vi "add_multi_controls_command.vi"(7 "Numeric":i32, 8 "error in":errorcluster, 9 "Controls Specs":T1[](array[typedef]), 10 "Instrument Command":string, 11 "VI Ref In":refnum<vi>) -> (0 "error out":errorcluster, 3 "VI Ref Out":refnum<vi>)   [LabVIEW 2018]
uses:
  TypeDefinitions/single_control_spec.ctl
  TypeDefinitions/control_data_type.ctl
  TypeDefinitions/control_class.ctl
  TypeDefinitions/ring_string_and_value.ctl
  Iternl/ConttWire/TypeDefines/connect_with_last_node_types.ctl
  Misc/AddNode/TypeDefinitions/node_types.ctl
  Iternl/GetNodeTerm/StringProcessingNode/TypeDefinitions/string_node_type.ctl
  Iternl/CalPos/CmdToStr/TypeDefinitions/main_position_types.ctl
  Iternl/AddObj/AddControl/TypeDefinitions/bd_control_type.ctl
  Iternl/CalPos/ParaToStr/TypeDefinitions/sub_position_type.ctl
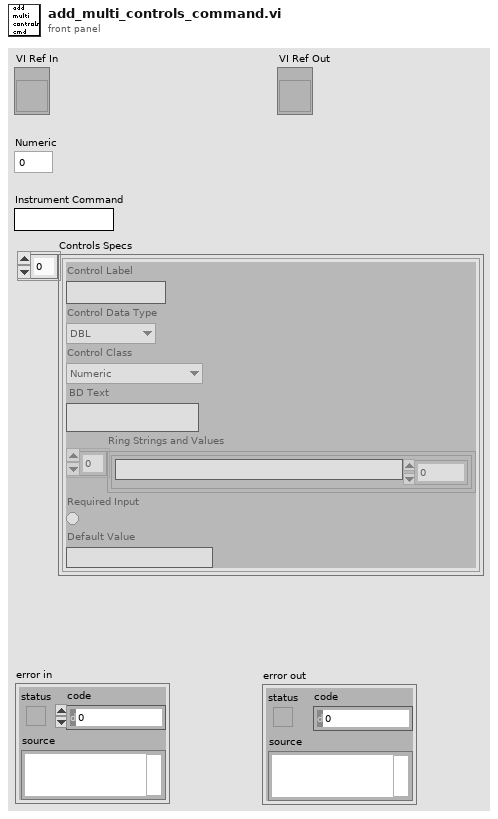
[diagram p1: front panel]
types:
  T1 = typedef "single_control_spec.ctl" = cluster{"Control Label":string, "Control Data Type":T2, "Control Class":T3, "BD Text":string, "Ring Strings and Values":T4[], "Required Input":bool, "Default Value":string}
  T2 = typedef "control_data_type.ctl" = enum16{"DBL", "I32", "Boolean", "String", "U16", "U32", "EXT", "SGL", "I16", "U8", "I8", "I64", "U64", "Waveform", "Reference", "Variant", "Cluster"}
  T3 = typedef "control_class.ctl" = enum16{"Numeric", "Vertical Slide Switch", "Text Ring", "String", "Array", "VISAName", "WaveformGraph", "Cluster"}
  T4 = typedef "ring_string_and_value.ctl" = cluster{"String":string, "Value":dbl}
  T5 = enum16{"Node", "FormatNodeForMultipleControls", "BoolConstant", "FormatConstant", "1stSubNodeX"}
  T6 = typedef "main_position_types.ctl" = enum16{"Node", "FormatNodeForMultipleControls", "BoolConstant", "FormatConstant", "1stSubNodeX"}
  T7 = typedef "string_node_type.ctl" = enum16{"FormatIntoString", "PickLine", "AppendTrueFalse", "ConcatenateStrings"}
  T8 = typedef "node_types.ctl" = enum16{"FormatIntoString", "PickLine", "AppendTrueFalse", "VISAWrite", "SubVI", "ConcatenateStrings", "VISARead", "ProperyNode", "ScanFromString", "SpreadSheetStringToArray"}
  T9 = typedef "sub_position_type.ctl" = enum16{"BoolNode", "BoolConst", "RingConstNode", "Numeri/String"}
  T10 = typedef "bd_control_type.ctl" = enum16{"Numeric", "Ring", "Boolean", "String", "VisaIn", "VisaOut", "Error In", "Error Out", "Array", "Waveform"}
  T11 = typedef "connect_with_last_node_types.ctl" = u16
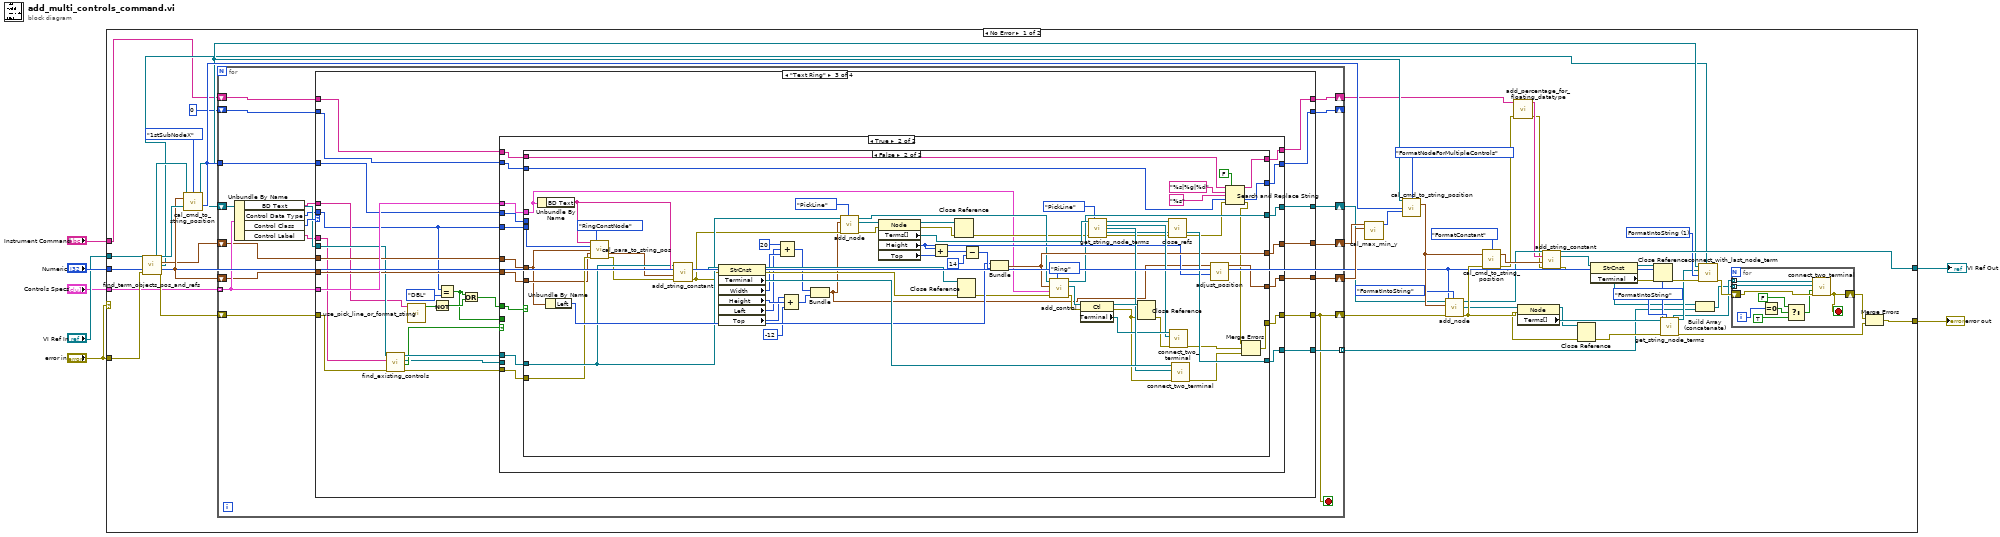
[diagram p0: block diagram]
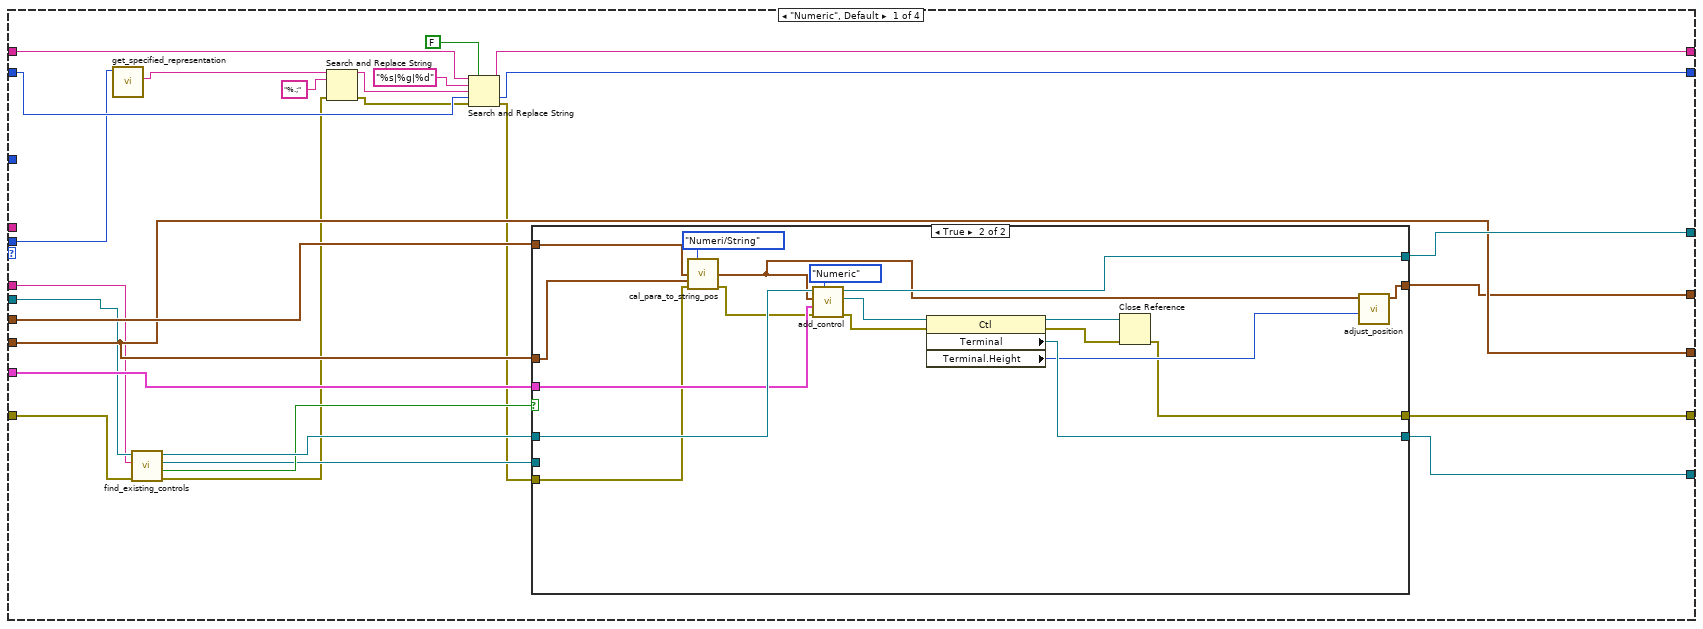
[diagram p2: hidden frame]
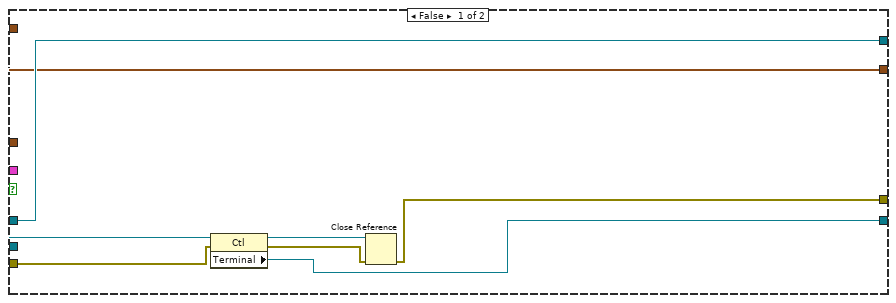
[diagram p3: hidden frame]
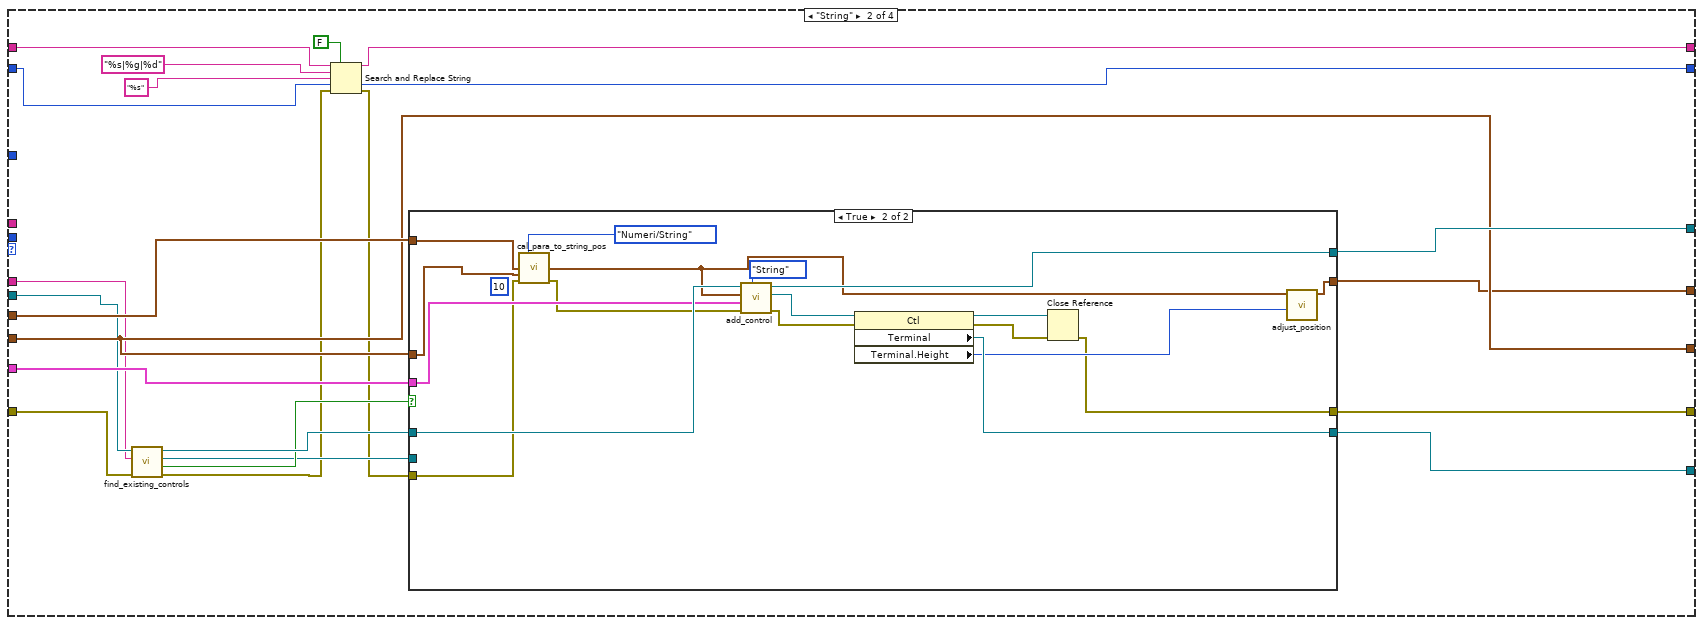
[diagram p4: hidden frame]
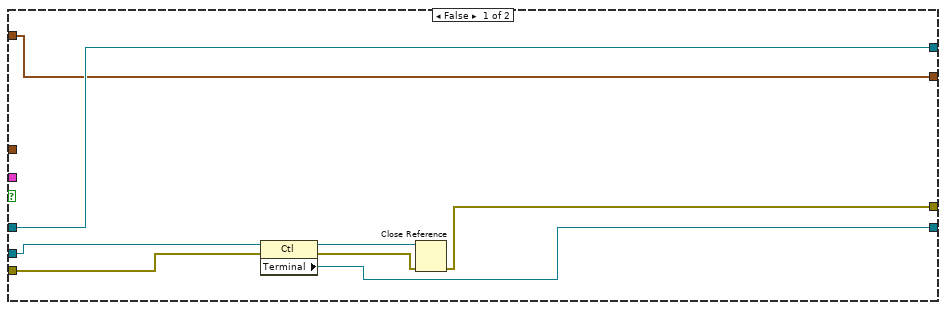
[diagram p5: hidden frame]
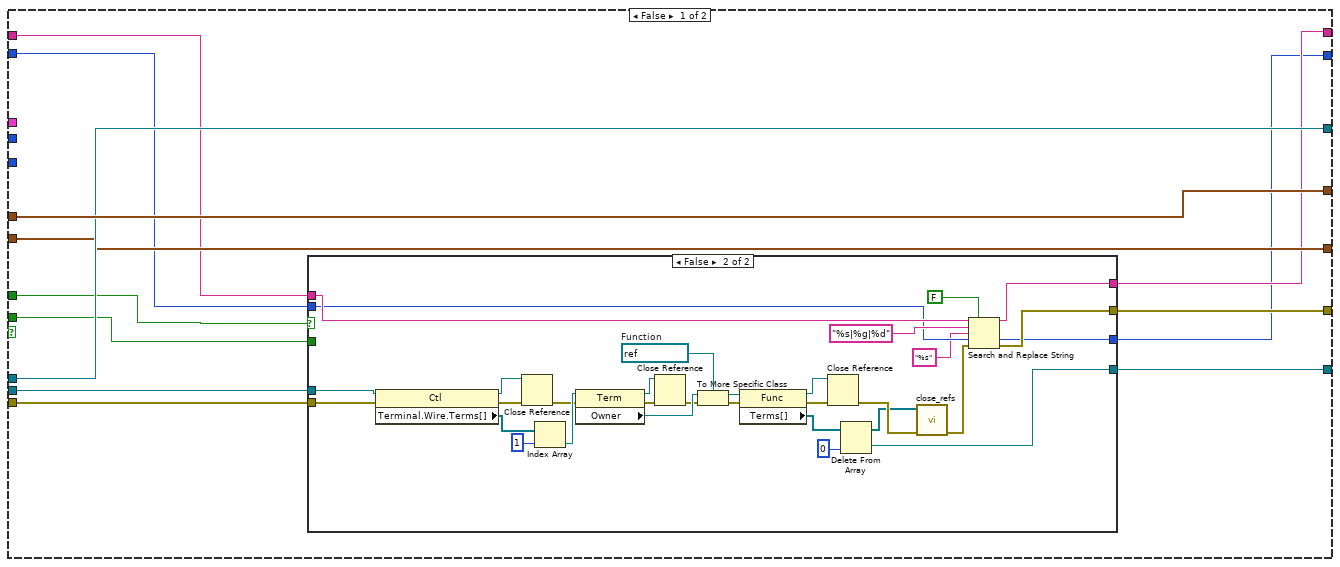
[diagram p6: hidden frame]
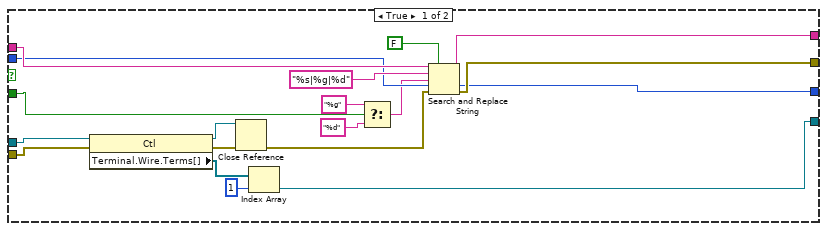
[diagram p7: hidden frame]
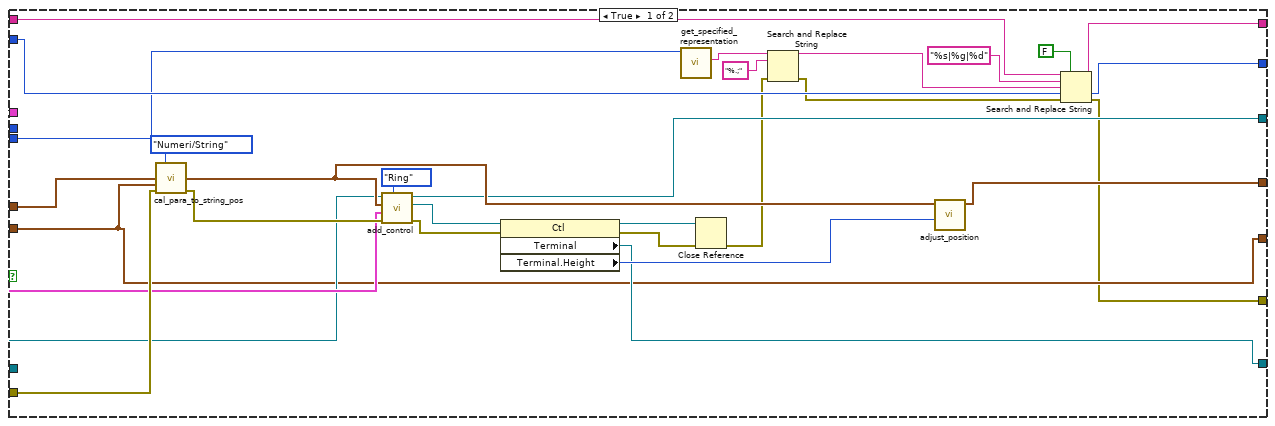
[diagram p8: hidden frame]
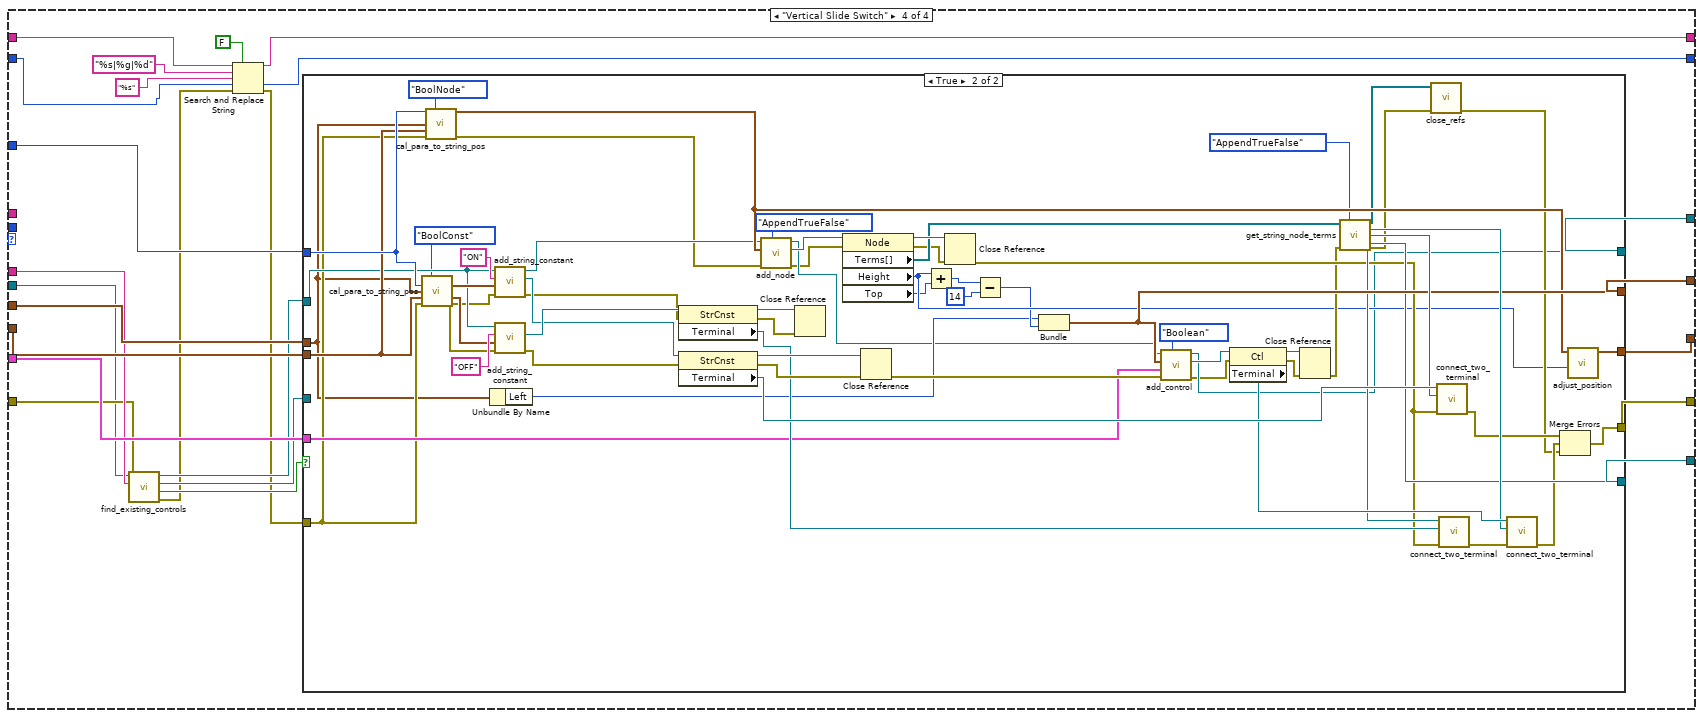
[diagram p9: hidden frame]
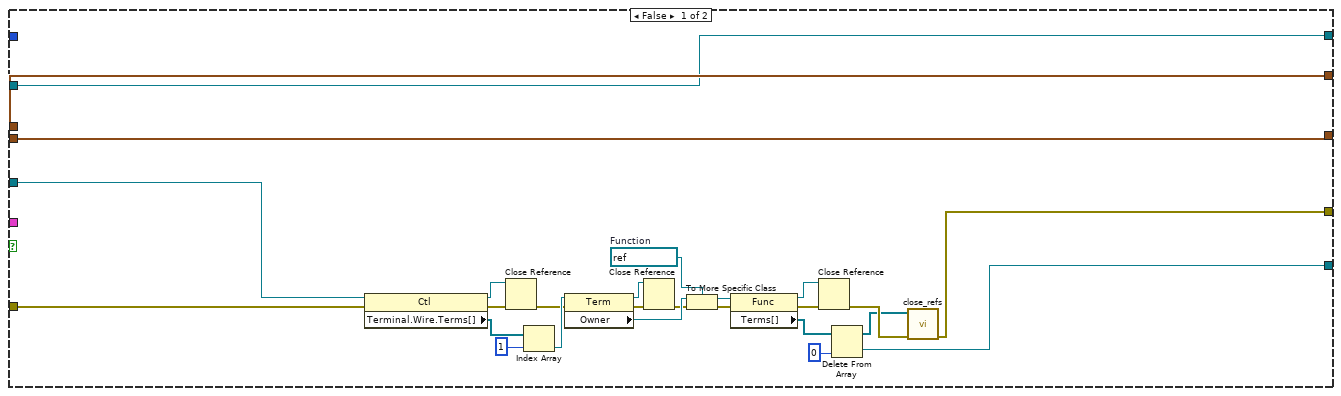
[diagram p10: hidden frame]
diagram:
  n1 = case shown="No Error" "error in" {
    tunnel: [w49 w506] -> w7
    tunnel: [w48 w507] -> w6
    tunnel: "error in" -> [w40 w507]
    tunnel: "Numeric" -> [w31 _]
    tunnel: "Instrument Command" -> [w13 _]
    tunnel: "VI Ref In" -> [w16 w506]
    tunnel: "Controls Specs" -> [w15 _]
    frame No Error {
      w34 = T11 1 items=["AppendTrueFalseString"=4, "PickLine"=3, "FormatIntoString"=1] ("Terminal Index")
      n2 = call "find_term_objects_pos_and_refs.vi"("VI Ref In"=w16, "error in (no error)"=w40) -> ("Last Function"=w38:refnum<vi>, "VI Ref Out"=w36:refnum<vi>, "Last Control Position"=w17:cluster{"Left":i32, "Top":i32}, "Last StrCnst Refnum"=w14:refnum<vi>, "Last Function Position"=w18:cluster{"Left":i32, "Top":i32}, "error out"=w41:errorcluster)  [unwired: 8 out]
      n3 = call "cal_cmd_to_string_position.vi"("Last Function Ref In"=w38, "Enum"=T5."1stSubNodeX", "Main Node BD Position"=w18) -> ("Last Function Ref Out"=w39:refnum<vi>, "1st sub node x position"=w56:i32)  [unwired: 4 in, 7 out]
      n4 = for {
        tunnel: w15 -> [w88] mode=indexing
        shift-right: [w85] -> w19
        shift-left: w36 -> [w86]
        tunnel: [w84] -> w25 mode=indexing
        shift-right: [w83] -> w58
        shift-left: w17 -> [w81]
        shift-right: [w80] -> w59
        shift-left: w18 -> [w82]
        tunnel: w56 -> [w79]
        shift-right: [w76] -> w42
        shift-left: w41 -> [w78]
        shift-right: [w73] -> w11
        shift-left: w13 -> [w75]
        shift-right: [w72] -> _
        shift-left: 0 -> [w74]
        stop <- w76 stop-if-true
        n5 = Unbundle By Name(w88) -> ("BD Text"=w70:string, "Control Data Type"=w71:T2, "Control Class"=w87:T3, "Control Label"=w77:string)
        n6 = case shown="\"Text Ring\"" w87 {
          tunnel: w88 -> [w114 w162 w215 w416]
          tunnel: w86 -> [w107 w155 w207 w404]
          tunnel: [w113 w161 w213 w415] -> w85
          tunnel: [w112 w160 w214 w413] -> w84
          tunnel: [w109 w157 w211 w414] -> w83
          tunnel: w82 -> [w110 w158 w209 w411]
          tunnel: w81 -> [w111 w159 w208 w412]
          tunnel: [w110 w158 w212 w410] -> w80
          tunnel: w79 -> [_ _ w210 w409]
          tunnel: w78 -> [w105 w153 w201 w406]
          tunnel: [w108 w156 w189 w408] -> w76
          tunnel: w77 -> [w106 w154 w204 w407]
          tunnel: w75 -> [w101 w143 w200 w395]
          tunnel: w74 -> [w99 w146 w199 w398]
          tunnel: [w89 w142 w198 w394] -> w73
          tunnel: [w90 w141 w197 w393] -> w72
          tunnel: w71 -> [w94 _ w194 _]
          tunnel: w70 -> [_ _ w196 _]
          frame "Numeric", Default {
            n7 = call "get_specified_representation.vi"("Control Data Type"=w94) -> ("Format String"=w96:string)  [unwired: 10 out]
            n8 = call "find_existing_controls.vi"("error in (no error)"=w105, "Label Text"=w106, "VI Ref In"=w107) -> ("error out"=w92:errorcluster, "New Ctrl"=w103:bool, "Ctrl Ref Out"=w102:refnum<vi>, "VI Ref Out"=w104:refnum<vi>)  [unwired: 5 out]
            n9 = Search and Replace String(input string=w96, search string="%.;", error in=w92) -> (result string=w93:string, error out=w91:errorcluster)  [unwired: 7 out]
            n10 = Search and Replace String(replace all?=FALSE ("replace all? (F)"), input string=w101, search string="%s|%g|%d", replace string=w93, offset=w99, error in=w91) -> (result string=w89:string, offset past replacement=w90:i32, error out=w97:errorcluster)  [unwired: 3 out]
            n11 = case shown="True" w103 {
              tunnel: w114 -> [_ w130]
              tunnel: [w120 w140] -> w113
              tunnel: [w116 w137] -> w112
              tunnel: w111 -> [w119 w128]
              tunnel: w110 -> [_ w127]
              tunnel: [w119 w133] -> w109
              tunnel: [w115 w132] -> w108
              tunnel: w97 -> [w121 w126]
              tunnel: w104 -> [w120 w131]
              tunnel: w102 -> [w122 _]
              frame False {
                n12 = property class="Ctl"(reference=w122, error in=w121) -> (reference out=w117:refnum<vi>, error out=w118:errorcluster, "Terminal"=w116:refnum<vi>)
                n13 = Close Reference(reference=w117, error in (no error)=w118) -> (error out=w115:errorcluster)
              }
              frame True {
                n14 = call "cal_para_to_string_pos.vi"("Enum"=sub_position_type."Numeri/String", "Last Control Position"=w128, "Last Function  Position"=w127, "error in"=w126) -> ("Control BD Position"=w125:cluster{"1st sub node x position":i32, i32}, "error out"=w124:errorcluster)  [unwired: 2 in, 8 out]
                n15 = call "add_control.vi"("Add Control Type"=bd_control_type."Numeric" ("Enum"), "error in (no error)"=w124, "Single Control Spec"=w130, "BD Position"=w125, "VI Ref In"=w131) -> ("error out"=w135:errorcluster, "Control Ref Out"=w139:refnum<vi>, "VI Ref Out"=w140:refnum<vi>)  [unwired: 4 out]
                n16 = property class="Ctl"(reference=w139, error in=w135) -> (reference out=w138:refnum<vi>, error out=w136:errorcluster, "Terminal"=w137:refnum<vi>, "Terminal.Height"=w134:u32)
                n17 = Close Reference(reference=w138, error in (no error)=w136) -> (error out=w132:errorcluster)
                n18 = call "adjust_position.vi"("Y Offset"=w134, "Position In"=w125) -> ("Position Out"=w133:cluster{"Left":i32, "Top":i32})  [unwired: 1 in, 8 out]
              }
            }
          }
          frame "String" {
            n19 = call "find_existing_controls.vi"("error in (no error)"=w153, "Label Text"=w154, "VI Ref In"=w155) -> ("error out"=w145:errorcluster, "New Ctrl"=w151:bool, "Ctrl Ref Out"=w150:refnum<vi>, "VI Ref Out"=w152:refnum<vi>)  [unwired: 5 out]
            n20 = Search and Replace String(replace all?=FALSE ("replace all? (F)"), input string=w143, search string="%s|%g|%d", replace string="%s" ("replace string (\"\")"), offset=w146, error in=w145) -> (result string=w142:string, offset past replacement=w141:i32, error out=w144:errorcluster)  [unwired: 3 out]
            n21 = case shown="True" w151 {
              tunnel: w162 -> [_ w178]
              tunnel: [w168 w188] -> w161
              tunnel: [w164 w185] -> w160
              tunnel: w159 -> [w167 w173]
              tunnel: w158 -> [_ w172]
              tunnel: [w167 w181] -> w157
              tunnel: [w163 w180] -> w156
              tunnel: w144 -> [w169 w175]
              tunnel: w152 -> [w168 w179]
              tunnel: w150 -> [w170 _]
              frame False {
                n22 = property class="Ctl"(reference=w170, error in=w169) -> (reference out=w165:refnum<vi>, error out=w166:errorcluster, "Terminal"=w164:refnum<vi>)
                n23 = Close Reference(reference=w165, error in (no error)=w166) -> (error out=w163:errorcluster)
              }
              frame True {
                (unwired) 10 ("y")
                n24 = call "cal_para_to_string_pos.vi"("Enum"=sub_position_type."Numeri/String", "Last Control Position"=w173, "Last Function  Position"=w172, "error in"=w175) -> ("Control BD Position"=w171:cluster{"1st sub node x position":i32, i32}, "error out"=w174:errorcluster)  [unwired: 2 in, 8 out]
                n25 = call "add_control.vi"("Add Control Type"=bd_control_type."String" ("Enum"), "error in (no error)"=w174, "Single Control Spec"=w178, "BD Position"=w171, "VI Ref In"=w179) -> ("error out"=w183:errorcluster, "Control Ref Out"=w187:refnum<vi>, "VI Ref Out"=w188:refnum<vi>)  [unwired: 4 out]
                n26 = property class="Ctl"(reference=w187, error in=w183) -> (reference out=w186:refnum<vi>, error out=w184:errorcluster, "Terminal"=w185:refnum<vi>, "Terminal.Height"=w182:u32)
                n27 = Close Reference(reference=w186, error in (no error)=w184) -> (error out=w180:errorcluster)
                n28 = call "adjust_position.vi"("Y Offset"=w182, "Position In"=w171) -> ("Position Out"=w181:cluster{"Left":i32, "Top":i32})  [unwired: 1 in, 8 out]
              }
            }
          }
          frame "Text Ring" {
            n29 = call "find_existing_controls.vi"("error in (no error)"=w201, "Label Text"=w204, "VI Ref In"=w207) -> ("error out"=w205:errorcluster, "New Ctrl"=w203:bool, "Ctrl Ref Out"=w202:refnum<vi>, "VI Ref Out"=w206:refnum<vi>)  [unwired: 5 out]
            n30 = call "use_pick_line_or_format_stirng.vi"("BD"=w196) -> ("Pick Line Node?"=w193:bool)  [unwired: 10 out]
            n31 = Not(x=w193) -> (.not. x?=w192:bool)
            n32 = Equal?(x=w194, y=control_data_type."DBL") -> (x = y?=w190:bool)
            n33 = Or(x=w190, y=w192) -> (x .or. y?=w191:bool)
            n34 = case shown="True" w203 {
              tunnel: w215 -> [_ w286]
              tunnel: [w222 w295] -> w214
              tunnel: [w227 w288] -> w213
              tunnel: [w226 w294] -> w212
              tunnel: [w228 w293] -> w211
              tunnel: w210 -> [_ w291]
              tunnel: w209 -> [w226 w287]
              tunnel: w208 -> [w228 w285]
              tunnel: [w225 w292] -> w189
              tunnel: w206 -> [w227 w290]
              tunnel: w205 -> [w223 w289]
              tunnel: w202 -> [w224 _]
              tunnel: w194 -> [_ w279]
              tunnel: w200 -> [w221 w283]
              tunnel: w199 -> [w220 w282]
              tunnel: [w219 w280] -> w198
              tunnel: [w218 w281] -> w197
              tunnel: w191 -> [w217 w284]
              tunnel: w190 -> [w216 _]
              frame False {
                n35 = case shown="False" w217 {
                  tunnel: [w231 w251] -> w225
                  tunnel: w224 -> [w244 w259]
                  tunnel: w223 -> [w243 w258]
                  tunnel: [w241 w257] -> w222
                  tunnel: w221 -> [w238 w254]
                  tunnel: w216 -> [w236 _]
                  tunnel: w220 -> [w237 w253]
                  tunnel: [w229 w249] -> w219
                  tunnel: [w230 w248] -> w218
                  frame True {
                    n36 = property class="Ctl"(reference=w244, error in=w243) -> (reference out=w242:refnum<vi>, error out=w247:errorcluster, "Terminal.Wire.Terms[]"=w246:refnum<vi>[])
                    n37 = Close Reference(reference=w242, error in (no error)=w247) -> (error out=w232:errorcluster)
                    n38 = Index Array(array=w246, index=1) -> (element=w241:refnum<vi>)
                    n39 = Select(t="%g", s=w236, f="%d" ("replace string (\"\")")) -> (s? t:f=w233:string)
                    n40 = Search and Replace String(replace all?=FALSE ("replace all? (F)"), input string=w238, search string="%s|%g|%d", replace string=w233, offset=w237, error in=w232) -> (result string=w229:string, offset past replacement=w230:i32, error out=w231:errorcluster)  [unwired: 3 out]
                  }
                  frame False {
                    w271 = refnum<vi> refnum  # Function
                    n41 = property class="Ctl"(reference=w259, error in=w258) -> (reference out=w270:refnum<vi>, error out=w269:errorcluster, "Terminal.Wire.Terms[]"=w276:refnum<vi>[])
                    n42 = Close Reference(reference=w270, error in (no error)=w269) -> (error out=w266:errorcluster)
                    n43 = Index Array(array=w276, index=1) -> (element=w277:refnum<vi>)
                    n44 = property class="Term"(reference=w277, error in=w266) -> (reference out=w268:refnum<vi>, error out=w267:errorcluster, "Owner"=w272:refnum<vi>)
                    n45 = Close Reference(reference=w268, error in (no error)=w267) -> (error out=w265:errorcluster)
                    n46 = To More Specific Class(target class=w271, reference=w272, error in=w265) -> (specific class reference=w275:refnum<vi>, error out=w273:errorcluster)
                    n47 = property class="Func"(reference=w275, error in=w273) -> (reference out=w262:refnum<vi>, error out=w264:errorcluster, "Terms[]"=w261:refnum<vi>[])
                    n48 = Close Reference(reference=w262, error in (no error)=w264) -> (error out=w263:errorcluster)
                    n49 = Delete From Array(array=w261, index=0) -> (deleted portion=w257:refnum<vi>, array with subset deleted=w260:refnum<vi>[])  [unwired: 1 in]
                    n50 = call "close_refs.vi"("error in"=w263, "Refs[]  In"=w260) -> ("error out"=w252:errorcluster)  [unwired: 9 out]
                    n51 = Search and Replace String(replace all?=FALSE ("replace all? (F)"), input string=w254, search string="%s|%g|%d", replace string="%s" ("replace string (\"\")"), offset=w253, error in=w252) -> (result string=w249:string, offset past replacement=w248:i32, error out=w251:errorcluster)  [unwired: 3 out]
                  }
                }
              }
              frame True {
                n52 = case shown="False" w284 {
                  tunnel: [w311 w379] -> w295
                  tunnel: [w309 w377] -> w294
                  tunnel: [w310 w376] -> w293
                  tunnel: [w304 w375] -> w292
                  tunnel: w291 -> [_ w374]
                  tunnel: w290 -> [w313 w365]
                  tunnel: w289 -> [w315 w363]
                  tunnel: [w312 w357] -> w288
                  tunnel: w287 -> [w309 w356]
                  tunnel: w286 -> [w314 w349]
                  tunnel: w285 -> [w316 w345]
                  tunnel: w283 -> [w306 w333]
                  tunnel: w282 -> [w305 w331]
                  tunnel: [w303 w328] -> w281
                  tunnel: [w302 w327] -> w280
                  tunnel: w279 -> [w299 _]
                  frame True {
                    n53 = call "cal_para_to_string_pos.vi"("Enum"=sub_position_type."Numeri/String", "Last Control Position"=w316, "Last Function  Position"=w309, "error in"=w315) -> ("Control BD Position"=w323:cluster{"1st sub node x position":i32, i32}, "error out"=w324:errorcluster)  [unwired: 2 in, 8 out]
                    n54 = call "add_control.vi"("Add Control Type"=bd_control_type."Ring" ("Enum"), "error in (no error)"=w324, "Single Control Spec"=w314, "BD Position"=w323, "VI Ref In"=w313) -> ("error out"=w320:errorcluster, "Control Ref Out"=w317:refnum<vi>, "VI Ref Out"=w312:refnum<vi>)  [unwired: 4 out]
                    n55 = property class="Ctl"(reference=w317, error in=w320) -> (reference out=w318:refnum<vi>, error out=w319:errorcluster, "Terminal"=w311:refnum<vi>, "Terminal.Height"=w321:u32)
                    n56 = call "get_specified_representation.vi"("Control Data Type"=w299) -> ("Format String"=w301:string)  [unwired: 10 out]
                    n57 = Close Reference(reference=w318, error in (no error)=w319) -> (error out=w298:errorcluster)
                    n58 = Search and Replace String(input string=w301, search string="%.;", error in=w298) -> (result string=w296:string, error out=w297:errorcluster)  [unwired: 7 out]
                    n59 = call "adjust_position.vi"("Y Offset"=w321, "Position In"=w323) -> ("Position Out"=w310:cluster{"Left":i32, "Top":i32})  [unwired: 1 in, 8 out]
                    n60 = Search and Replace String(replace all?=FALSE ("replace all? (F)"), input string=w306, search string="%s|%g|%d", replace string=w296, offset=w305, error in=w297) -> (result string=w302:string, offset past replacement=w303:i32, error out=w304:errorcluster)  [unwired: 3 out]
                  }
                  frame False {
                    n61 = Unbundle By Name(w349) -> ("BD Text"=w370:string)
                    n62 = Unbundle By Name(w345) -> ("Left"=w366:i32)
                    n63 = call "cal_para_to_string_pos.vi"("Bool Disable Command"=w370, "Enum"=sub_position_type."RingConstNode", "1st sub node x position"=w374, "Last Control Position"=w345, "Last Function  Position"=w356, "error in"=w363) -> ("BD Constant Position/Disable String Position"=w326:cluster{"1st sub node x position":i32, i32}, "error out"=w360:errorcluster)  [unwired: 8 out]
                    n64 = call "add_string_constant.vi"("error in"=w360, "BD Position"=w326, "StringConstantValue"=w370, "VI Ref In"=w365) -> ("error out"=w362:errorcluster, "StrCnst Refnum"=w373:refnum<vi>)  [unwired: 6 out]
                    n65 = property class="StrCnst"(reference=w373, error in=w362) -> (reference out=w392:refnum<vi>, error out=w378:errorcluster, "Terminal"=w383:refnum<vi>, "Width"=w344:u32, "Height"=w342:u32, "Left"=w338:i32, "Top"=w337:i32)
                    n66 = Compound Arithmetic op=ADD(20 ("value"), w338, w344) -> (w340:u32)
                    n67 = Compound Arithmetic op=ADD(w337, w342, -12 ("value")) -> (w339:u32)
                    n68 = Bundle(w340, w339) -> (w336:cluster{u32, u32})  [unwired: 1 out]
                    n69 = call "add_node.vi"("Node Type"=node_types."PickLine" ("Enum"), "error in (no error)"=w362, "BD Position"=w336, "VI Ref In"=w365) -> ("error out"=w361:errorcluster, "Node Refnum"=w391:refnum<vi>, "VI Ref Out"=w358:refnum<vi>)  [unwired: 2 in, 3 out]
                    n70 = property class="Node"(reference=w391, error in=w361) -> (reference out=w387:refnum<vi>, error out=w386:errorcluster, "Terms[]"=w385:refnum<vi>[], "Height"=w372:u32, "Top"=w371:i32)
                    n71 = Add(x=w372, y=w371) -> (x+y=w369:u32)
                    n72 = Close Reference(reference=w387, error in (no error)=w386) -> (error out=w352:errorcluster)
                    n73 = Close Reference(reference=w392, error in (no error)=w378) -> (error out=w359:errorcluster)
                    n74 = Subtract(x=w369, y=u32 14) -> (x-y=w367:u32)
                    n75 = Bundle("Left"=w366, w367) -> (w376:cluster{"Left":i32, u32})  [unwired: 1 out]
                    n76 = call "add_control.vi"("Add Control Type"=bd_control_type."Ring" ("Enum"), "error in (no error)"=w359, "Single Control Spec"=w349, "BD Position"=w376, "VI Ref In"=w358) -> ("error out"=w389:errorcluster, "Control Ref Out"=w390:refnum<vi>, "VI Ref Out"=w357:refnum<vi>)  [unwired: 4 out]
                    n77 = property class="Ctl"(reference=w390, error in=w389) -> (reference out=w388:refnum<vi>, error out=w355:errorcluster, "Terminal"=w381:refnum<vi>)
                    n78 = call "get_string_node_terms.vi"("Terms[] In"=w385, "Node Type"=string_node_type."PickLine", "error in (no error)"=w352) -> ("Terms[]  Out"=w384:refnum<vi>[], "Pick Term"=w380:refnum<vi>, "Multiline Term/Enable Term/Concantenate Term"=w382:refnum<vi>, "Pick Line Output Term/Disable Term"=w379:refnum<vi>, "error out"=w351:errorcluster)  [unwired: 1 in, 7 out]
                    n79 = Close Reference(reference=w388, error in (no error)=w355) -> (error out=w364:errorcluster)
                    n80 = call "close_refs.vi"("error in"=w351, "Refs[]  In"=w384) -> ("error out"=w330:errorcluster)  [unwired: 9 out]
                    n81 = call "connect_two_terminal.vi"("error in"=w364, "Terminal 2"=w380, "Terminal 1"=w381) -> ("error out"=w354:errorcluster)  [unwired: 1 in, 7 out]
                    n82 = call "connect_two_terminal.vi"("error in"=w355, "Terminal 2"=w382, "Terminal 1"=w383) -> ("error out"=w353:errorcluster)  [unwired: 1 in, 7 out]
                    n83 = call "adjust_position.vi"("Y Offset"=w372, "Position In"=w336) -> ("Position Out"=w377:cluster{"Left":i32, "Top":i32})  [unwired: 1 in, 8 out]
                    n84 = Search and Replace String(replace all?=FALSE ("replace all? (F)"), input string=w333, search string="%s|%g|%d", replace string="%s" ("replace string (\"\")"), offset=w331, error in=w330) -> (result string=w327:string, offset past replacement=w328:i32, error out=w329:errorcluster)  [unwired: 3 out]
                    n85 = Merge Errors(w329, w354, w353) -> (w375:errorcluster)
                  }
                }
              }
            }
          }
          frame "Vertical Slide Switch" {
            n86 = call "find_existing_controls.vi"("error in (no error)"=w406, "Label Text"=w407, "VI Ref In"=w404) -> ("error out"=w397:errorcluster, "New Ctrl"=w405:bool, "Ctrl Ref Out"=w402:refnum<vi>, "VI Ref Out"=w403:refnum<vi>)  [unwired: 5 out]
            n87 = Search and Replace String(replace all?=FALSE ("replace all? (F)"), input string=w395, search string="%s|%g|%d", replace string="%s" ("replace string (\"\")"), offset=w398, error in=w397) -> (result string=w394:string, offset past replacement=w393:i32, error out=w396:errorcluster)  [unwired: 3 out]
            n88 = case shown="True" w405 {
              tunnel: w416 -> [_ w463]
              tunnel: [w417 w470] -> w415
              tunnel: [w418 w495] -> w414
              tunnel: [w420 w492] -> w413
              tunnel: w412 -> [w418 w443]
              tunnel: w411 -> [w419 w459]
              tunnel: [w419 w487] -> w410
              tunnel: w409 -> [_ w460]
              tunnel: [w421 w481] -> w408
              tunnel: w403 -> [w417 w451]
              tunnel: w396 -> [w422 w445]
              tunnel: w402 -> [w423 _]
              frame False {
                w435 = refnum<vi> refnum  # Function
                n89 = property class="Ctl"(reference=w423, error in=w422) -> (reference out=w434:refnum<vi>, error out=w433:errorcluster, "Terminal.Wire.Terms[]"=w440:refnum<vi>[])
                n90 = Close Reference(reference=w434, error in (no error)=w433) -> (error out=w430:errorcluster)
                n91 = Index Array(array=w440, index=1) -> (element=w441:refnum<vi>)
                n92 = property class="Term"(reference=w441, error in=w430) -> (reference out=w432:refnum<vi>, error out=w431:errorcluster, "Owner"=w436:refnum<vi>)
                n93 = Close Reference(reference=w432, error in (no error)=w431) -> (error out=w429:errorcluster)
                n94 = To More Specific Class(target class=w435, reference=w436, error in=w429) -> (specific class reference=w439:refnum<vi>, error out=w437:errorcluster)
                n95 = property class="Func"(reference=w439, error in=w437) -> (reference out=w426:refnum<vi>, error out=w428:errorcluster, "Terms[]"=w425:refnum<vi>[])
                n96 = Close Reference(reference=w426, error in (no error)=w428) -> (error out=w427:errorcluster)
                n97 = Delete From Array(array=w425, index=0) -> (deleted portion=w420:refnum<vi>, array with subset deleted=w424:refnum<vi>[])  [unwired: 1 in]
                n98 = call "close_refs.vi"("error in"=w427, "Refs[]  In"=w424) -> ("error out"=w421:errorcluster)  [unwired: 9 out]
              }
              frame True {
                n99 = call "cal_para_to_string_pos.vi"("Enum"=sub_position_type."BoolConst", "1st sub node x position"=w460, "Last Control Position"=w443, "Last Function  Position"=w459, "error in"=w445) -> ("Bool Node BD Position/Enable String Position"=w452:cluster{"1st sub node x position":i32, i32}, "BD Constant Position/Disable String Position"=w453:cluster{"1st sub node x position":i32, i32}, "error out"=w448:errorcluster)  [unwired: 1 in, 7 out]
                n100 = call "cal_para_to_string_pos.vi"("Enum"=sub_position_type."BoolNode", "1st sub node x position"=w460, "Last Control Position"=w443, "Last Function  Position"=w459, "error in"=w445) -> ("Bool Node BD Position/Enable String Position"=w488:cluster{"1st sub node x position":i32, i32}, "error out"=w447:errorcluster)  [unwired: 1 in, 8 out]
                n101 = Unbundle By Name(w443) -> ("Left"=w473:i32)
                n102 = call "add_string_constant.vi"("error in"=w448, "BD Position"=w452, "StringConstantValue"="ON", "VI Ref In"=w451) -> ("error out"=w450:errorcluster, "StrCnst Refnum"=w454:refnum<vi>, "VI Ref Out"=w456:refnum<vi>)  [unwired: 5 out]
                n103 = call "add_string_constant.vi"("error in"=w448, "BD Position"=w453, "StringConstantValue"="OFF", "VI Ref In"=w451) -> ("error out"=w449:errorcluster, "StrCnst Refnum"=w455:refnum<vi>)  [unwired: 6 out]
                n104 = property class="StrCnst"(reference=w455, error in=w450) -> (reference out=w494:refnum<vi>, error out=w493:errorcluster, "Terminal"=w490:refnum<vi>)
                n105 = property class="StrCnst"(reference=w454, error in=w449) -> (reference out=w505:refnum<vi>, error out=w496:errorcluster, "Terminal"=w500:refnum<vi>)
                n106 = call "add_node.vi"("Node Type"=node_types."AppendTrueFalse" ("Enum"), "error in (no error)"=w447, "BD Position"=w488, "VI Ref In"=w456) -> ("error out"=w468:errorcluster, "Node Refnum"=w504:refnum<vi>, "VI Ref Out"=w471:refnum<vi>)  [unwired: 2 in, 3 out]
                n107 = Close Reference(reference=w494, error in (no error)=w493) -> ()  [unwired: 1 out]
                n108 = property class="Node"(reference=w504, error in=w468) -> (reference out=w501:refnum<vi>, error out=w467:errorcluster, "Terms[]"=w472:refnum<vi>[], "Height"=w478:u32, "Top"=w477:i32)
                n109 = Close Reference(reference=w505, error in (no error)=w496) -> (error out=w485:errorcluster)
                n110 = Add(x=w478, y=w477) -> (x+y=w476:u32)
                n111 = Close Reference(reference=w501, error in (no error)=w467) -> (error out=w486:errorcluster)
                n112 = Subtract(x=w476, y=u32 14) -> (x-y=w474:u32)
                n113 = Bundle("Left"=w473, w474) -> (w495:cluster{"Left":i32, u32})  [unwired: 1 out]
                n114 = call "add_control.vi"("Add Control Type"=bd_control_type."Boolean" ("Enum"), "error in (no error)"=w485, "Single Control Spec"=w463, "BD Position"=w495, "VI Ref In"=w471) -> ("error out"=w465:errorcluster, "Control Ref Out"=w503:refnum<vi>, "VI Ref Out"=w470:refnum<vi>)  [unwired: 4 out]
                n115 = property class="Ctl"(reference=w503, error in=w465) -> (reference out=w502:refnum<vi>, error out=w466:errorcluster, "Terminal"=w498:refnum<vi>)
                n116 = Close Reference(reference=w502, error in (no error)=w466) -> (error out=w484:errorcluster)
                n117 = call "get_string_node_terms.vi"("Terms[] In"=w472, "Node Type"=string_node_type."AppendTrueFalse", "error in (no error)"=w484) -> ("Terms[]  Out"=w480:refnum<vi>[], "Pick Term"=w497:refnum<vi>, "Multiline Term/Enable Term/Concantenate Term"=w499:refnum<vi>, "Pick Line Output Term/Disable Term"=w491:refnum<vi>, "Bool Output Term"=w492:refnum<vi>, "error out"=w469:errorcluster)  [unwired: 1 in, 6 out]
                n118 = call "close_refs.vi"("error in"=w469, "Refs[]  In"=w480) -> ("error out"=w479:errorcluster)  [unwired: 9 out]
                n119 = call "connect_two_terminal.vi"("error in"=w486, "Terminal 2"=w499, "Terminal 1"=w500) -> ("error out"=w483:errorcluster)  [unwired: 1 in, 7 out]
                n120 = call "connect_two_terminal.vi"("error in"=w486, "Terminal 2"=w490, "Terminal 1"=w491) -> ("error out"=w489:errorcluster)  [unwired: 1 in, 7 out]
                n121 = call "connect_two_terminal.vi"("error in"=w489, "Terminal 2"=w497, "Terminal 1"=w498) -> ("error out"=w482:errorcluster)  [unwired: 1 in, 7 out]
                n122 = Merge Errors(w483, w482, w479) -> (w481:errorcluster)
                n123 = call "adjust_position.vi"("Y Offset"=w478, "Position In"=w488) -> ("Position Out"=w487:cluster{"Left":i32, "Top":i32})  [unwired: 1 in, 8 out]
              }
            }
          }
        }
      }
      n124 = call "cal_max_min_y.vi"("Position 2"=w59, "Position 1"=w58) -> ("max y"=w60:i32)  [unwired: 9 out]
      n125 = call "cal_cmd_to_string_position.vi"("Last Function Ref In"=w39, "Enum"=main_position_types."FormatNodeForMultipleControls", "1st sub node x position"=w56, "Last sub node y position/Offset"=w60) -> ("Main Node Position/Enable Constant Position"=w52:cluster{"Left":u32, "Top":i32})  [unwired: 3 in, 8 out]
      n126 = call "add_node.vi"("Node Type"=node_types."FormatIntoString" ("Enum"), "error in (no error)"=w42, "Number of Parameters"=w31, "BD Position"=w52, "VI Ref In"=w19) -> ("error out"=w43:errorcluster, "Node Refnum"=w27:refnum<vi>, "VI Ref Out"=w20:refnum<vi>)  [unwired: 1 in, 3 out]
      n127 = call "cal_cmd_to_string_position.vi"("Enum"=main_position_types."FormatConstant", "Main Node BD Position"=w52, "error in (no error)"=w43) -> ("Main Node Position/Enable Constant Position"=w53:cluster{"Left":u32, "Top":i32}, "error out"=w9:errorcluster)  [unwired: 4 in, 7 out]
      n128 = call "add_percentage_for_floating_datatype.vi"("error in (no error)"=w9, "String In"=w11) -> ("error out"=w8:errorcluster, "String Out"=w10:string)  [unwired: 8 out]
      n129 = property class="Node"(reference=w27, error in=w43) -> (reference out=w28:refnum<vi>, error out=w29:errorcluster, "Terms[]"=w30:refnum<vi>[])
      n130 = call "add_string_constant.vi"("error in"=w8, "BD Position"=w53, "StringConstantValue"=w10, "VI Ref In"=w20) -> ("error out"=w22:errorcluster, "StrCnst Refnum"=w21:refnum<vi>, "VI Ref Out"=w49:refnum<vi>)  [unwired: 5 out]
      n131 = Close Reference(reference=w28, error in (no error)=w29) -> (error out=w44:errorcluster)
      n132 = property class="StrCnst"(reference=w21, error in=w22) -> (reference out=w23:refnum<vi>, error out=w45:errorcluster, "Terminal"=w24:refnum<vi>)
      n133 = Close Reference(reference=w23, error in (no error)=w45) -> (error out=w37:errorcluster)
      n134 = call "get_string_node_terms.vi"("Terms[] In"=w30, "Node Type"=string_node_type."FormatIntoString", "Number of Parameters"=w31, "error in (no error)"=w44) -> ("Format Terms Out"=w32:refnum<vi>[], "Terms[]  Out"=w33:refnum<vi>[], "error out"=w47:errorcluster)  [unwired: 9 out]
      n135 = Build Array (concatenate)(w24, w25) -> (w26:refnum<vi>[])
      n136 = call "connect_with_last_node_term.vi"("Last StrCnst Refnum"=w14, "error in (no error)"=w37, "Terminal Index"=w34, "Terminals[]"=w33, "Last Function Ref In"=w39) -> ("error out"=w35:errorcluster)  [unwired: 6 out]
      n137 = for {
        shift-right: [w61] -> w46
        shift-left: w35 -> [w69]
        tunnel: w26 -> [w67] mode=indexing
        tunnel: w32 -> [w68] mode=indexing
        i -> [w64]
        stop <- w61 stop-if-true
        n138 = Equal To 0?(x=w64) -> (x = 0?=w66:bool)
        n139 = Select(t=FALSE ("Auto Route? (T)"), s=w66, f=TRUE ("Auto Route? (T)")) -> (s? t:f=w63:bool)
        n140 = call "connect_two_terminal.vi"("error in"=w69, "Auto Route? (T)"=w63, "Terminal 2"=w67, "Terminal 1"=w68) -> ("error out"=w61:errorcluster)  [unwired: 7 out]
      }
      n141 = Merge Errors(w46, w47) -> (w48:errorcluster)
    }
    frame Error {
    }
  }
  "VI Ref Out" <- w7
  "error out" <- w6
